vi "LabS3_Probe1_Ejercicio.vi"() -> ()   [LabVIEW 2012]
panel:
  in  "Numeric":dbl
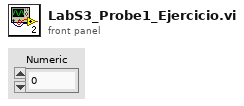
[diagram p1: front panel]
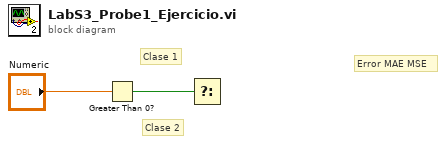
[diagram p0: block diagram]
diagram:
  # "Clase 2"
  # "Clase 1"
  # "Error MAE MSE"
  n1 = Greater Than 0?(x="Numeric") -> (x > 0?=w1:bool)
  n2 = Select(s=w1) -> ()  [unwired: 2 in, 1 out]
